vi "ma_Averaged DC-RMS no State.vi"(0 "signal in":waveform(dbl), 1 "reset":bool, 5 "averaging type":enum16{"Linear", "Exponential"}(ring), 7 "state info":T1 {"buffer" format="%0.2f"; "timestamp" format="%<%.4X>T"; "dt history" format="%0.2f"; "t0 history" format="%<%I:%M:%S%4u %p>T"; "exp TC (samples)" format="%0.2f"; "RMS history" format="%0.2f"; "DC history" format="%0.2f"}, 9 "averaging time":dbl=-1.0 format="%0.2p", 11 "error in":errorcluster, 12 "averaging control":T3={"window for DC"=enum."Rectangular (none)", "output function"=enum."DC and RMS", "window for RMS"=enum."Rectangular (none)", "exp. time constant"=-1.0, "Ignore input start time"=FALSE} {"exp. time constant" format="%0.2p"}) -> (3 "data ready":bool, 4 "DC value waveform":waveform(dbl), 6 "RMS value waveform":waveform(dbl), 8 "state info":T1 {"buffer" format="%0.2f"; "timestamp" format="%<%.4X>T"; "dt history" format="%0.2f"; "t0 history" format="%<%I:%M:%S%4u %p>T"; "exp TC (samples)" format="%0.2f"; "RMS history" format="%0.2f"; "DC history" format="%0.2f"}, 14 "measurement info cluster":T2={"uncertainty"=0.0, "Warning"=FALSE, "comments"="reserved for future use"} {"uncertainty" format="%0.2p"}, 15 "error out":errorcluster)   [LabVIEW 2020, in "NI_MAPro.lvlib"]
doc: "This VI calculates the DC and/or the RMS values of an input waveform. This VI gives more precise control over the individual calculations (DC and/or RMS) than the Basic Averaged DC-RMS VI. The outputs are waveforms that show the current and past DC and RMS values calculated."
uses:
  NI_MAPro.lvlib
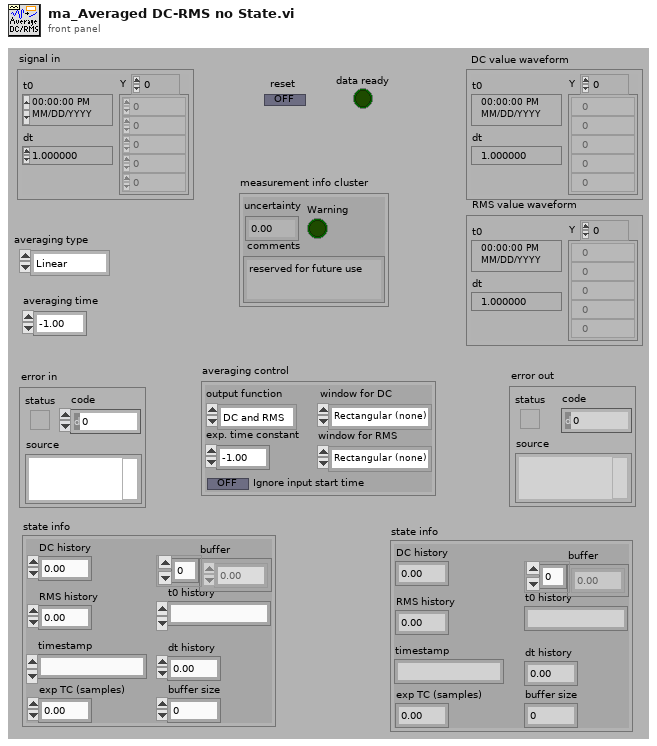
[diagram p1: front panel]
types:
  T1 = cluster{"DC history":dbl, "RMS history":dbl, "exp TC (samples)":dbl, "buffer size":i32, "t0 history":timestamp, "dt history":dbl, "timestamp":timestamp, "buffer":dbl[]}
  T2 = cluster{"uncertainty":dbl, "Warning":bool, "comments":string}
  T3 = cluster{"window for DC":enum16{"Rectangular (none)", "Hanning", "Low side lobe"}, "output function":enum16{"DC only", "RMS only", "DC and RMS"}, "window for RMS":enum16{"Rectangular (none)", "Hanning", "Low side lobe"}, "exp. time constant":dbl, "Ignore input start time":bool}
  T4 = enum16{"Rectangular (none)", "Hanning", "Low side lobe"}
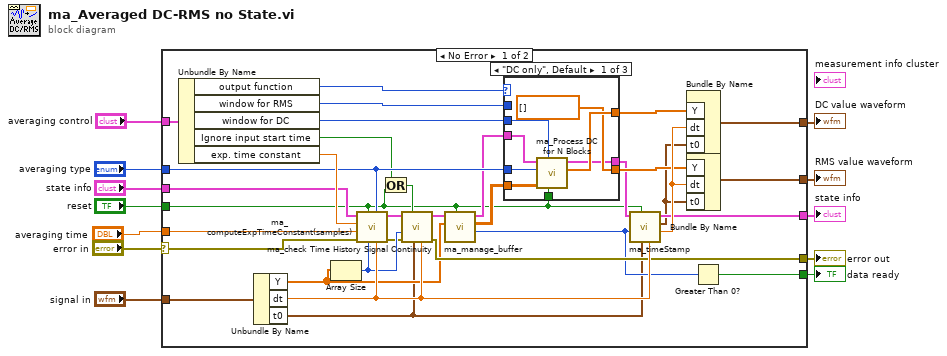
[diagram p0: block diagram]
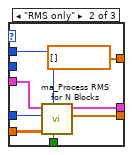
[diagram p2: hidden frame]
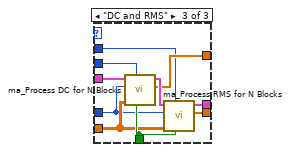
[diagram p3: hidden frame]
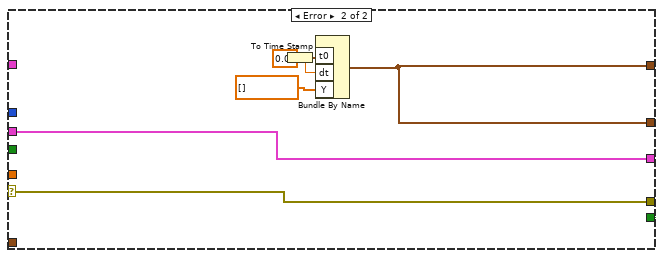
[diagram p4: hidden frame]
diagram:
  n1 = case shown="No Error" "error in" {
    selector: "error in" -> [w36 w75]
    tunnel: [w35 w75] -> w12
    tunnel: [w42 w76] -> w10
    tunnel: [w41 w76] -> w11
    tunnel: "reset" -> [w13 _]
    tunnel: "averaging time" -> [w40 _]
    tunnel: "signal in" -> [w39 _]
    tunnel: "averaging control" -> [w34 _]
    tunnel: [w38 FALSE] -> w5
    tunnel: "averaging type" -> [w37 _]
    tunnel: "state info" -> [w21 w73]
    tunnel: [w33 w73] -> w2
    frame No Error {
      n2 = Unbundle By Name(w34) -> ("output function"=w20:enum16{"DC only", "RMS only", "DC and RMS"}, "window for RMS"=w19:T4, "window for DC"=w18:T4, "Ignore input start time"=w14:bool, "exp. time constant"=w45:dbl)
      n3 = Unbundle By Name(w39) -> ("Y"=w30:dbl[], "dt"=w43:dbl, "t0"=w17:timestamp)
      n4 = Array Size(array=w30) -> (size(s)=w32:i32)
      n5 = call "ma_computeExpTimeConstant(samples).vi"("dt"=w43, "averaging type"=w37, "num Points"=w32, "reset"=w13, "error in (no error)"=w36, "averaging time"=w40, "exp. time constant"=w45, "state info"=w21) -> ("error out"=w29:errorcluster, "state info"=w28:T1)  [unwired: 2 in]
      n6 = Or(x=w14, y=w13) -> (x .or. y?=w15:bool)
      n7 = call "ma_check Time History Signal Continuity.vi"("dt"=w43, "t0"=w17, "Ignore input start time"=w15, "error in (no error)"=w29, "# samples"=w32, "state info"=w28) -> ("error out"=w35:errorcluster, "state info"=w27:T1)  [unwired: 1 in, 3 out]
      n8 = call "ma_manage_buffer.vi"("Initialize"=w13, "Y"=w30, "state info"=w27) -> ("#blocks"=w31:i32, "Output Array"=w26:dbl[][], "state info"=w23:T1)  [unwired: 6 in]
      n9 = case shown="\"DC only\", Default" w20 {
        tunnel: w26 -> [w53 w60 w70]
        tunnel: w23 -> [w52 w61 w66]
        tunnel: w13 -> [w51 w59 w71]
        tunnel: [w50 dbl[] [] ("DC value data") w64] -> w24
        tunnel: [w48 w57 w68] -> w22
        tunnel: w37 -> [w47 w54 w65]
        tunnel: w19 -> [_ w58 w63]
        tunnel: [dbl[] [] ("RMS value data") w56 w67] -> w25
        tunnel: w18 -> [w46 _ w62]
        frame "DC only", Default {
          n10 = call "ma_Process DC for N Blocks.vi"("reset"=w51, "window for DC"=w46, "time signal data (samples)"=w53, "averaging type"=w47, "state info"=w52) -> ("DC value data"=w50:dbl[], "state info"=w48:T1)  [unwired: 5 in]
        }
        frame "RMS only" {
          n11 = call "ma_Process RMS for N Blocks.vi"("reset"=w59, "window for RMS"=w58, "time signal data (samples)"=w60, "averaging type"=w54, "state info"=w61) -> ("RMS value data"=w56:dbl[], "state info"=w57:T1)  [unwired: 5 in]
        }
        frame "DC and RMS" {
          n12 = call "ma_Process DC for N Blocks.vi"("reset"=w71, "window for DC"=w62, "time signal data (samples)"=w70, "averaging type"=w65, "state info"=w66) -> ("DC value data"=w64:dbl[], "state info"=w69:T1)  [unwired: 5 in]
          n13 = call "ma_Process RMS for N Blocks.vi"("reset"=w71, "window for RMS"=w63, "time signal data (samples)"=w70, "averaging type"=w65, "state info"=w69) -> ("RMS value data"=w67:dbl[], "state info"=w68:T1)  [unwired: 5 in]
        }
      }
      n14 = call "ma_timeStamp.vi"("dt"=w43, "t0"=w17, "reset"=w13, "Number of blocks"=w31, "state info"=w22) -> ("dt"=w44:dbl, "t0"=w16:timestamp, "state info"=w33:T1)  [unwired: 4 in]
      n15 = Bundle By Name("Y"=w24, "dt"=w44, "t0"=w16) -> (w41:waveform(dbl))  [unwired: 1 in]
      n16 = Bundle By Name("Y"=w25, "dt"=w44, "t0"=w16) -> (w42:waveform(dbl))  [unwired: 1 in]
      n17 = Greater Than 0?(x=w31) -> (x > 0?=w38:bool)
    }
    frame Error {
      w78 = 0.0 ("t0")
      n18 = To Time Stamp(1:w78) -> (0:w72:timestamp)
      n19 = Bundle By Name("t0"=w72, "dt"=w78, "Y"=dbl[] [] ("DC value data")) -> (w76:waveform(dbl))  [unwired: 1 in]
    }
  }
  "error out" <- w12
  "DC value waveform" <- w11
  "RMS value waveform" <- w10
  "data ready" <- w5
  "state info" <- w2
